vi "Array to Wfm (N Ch).vi"(8 "channel names":string[](array[string]), 10 "dt":dbl, 11 "array":dbl[](array[numeric])) -> (3 "waveforms":waveform(dbl)[](array[waveform]))   [LabVIEW 2023]
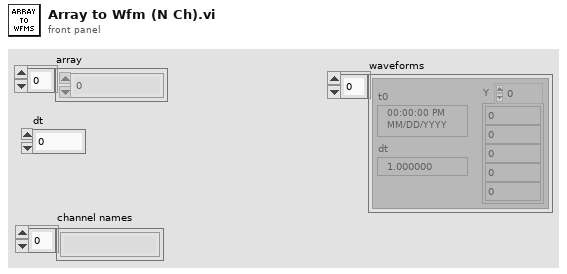
[diagram p1: front panel]
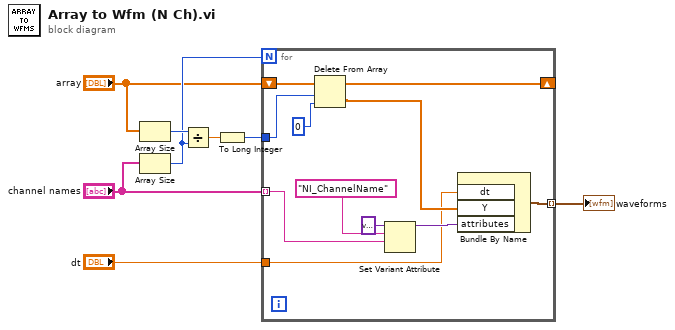
[diagram p0: block diagram]
diagram:
  n1 = Array Size(array="array") -> (size(s)=w8:i32)
  n2 = Array Size(array="channel names") -> (size(s)=w7:i32)
  n3 = Divide(x=w8, y=w7) -> (x/y=w5:dbl)
  n4 = To Long Integer(number=w5) -> (32bit integer=w4:i32)
  n5 = for {
    N: w7 -> [_]
    shift-right: [w18] -> _
    shift-left: "array" -> [w19]
    tunnel: w4 -> [w16]
    tunnel: "channel names" -> [w12] mode=indexing
    tunnel: "dt" -> [w13]
    tunnel: [w10] -> w1 mode=indexing
    n6 = Delete From Array(array=w19, length=w16, index=0) -> (deleted portion=w14:dbl[], array with subset deleted=w18:dbl[])
    n7 = Set Variant Attribute(Variant=variant ("variant"), name="NI_ChannelName", value=w12) -> (Variant out=w15:variant)  [unwired: 1 in, 2 out]
    n8 = Bundle By Name("dt"=w13, "Y"=w14, "attributes"=w15) -> (w10:waveform(dbl))  [unwired: 1 in]
  }
  "waveforms" <- w1
